vi "Handle Error.vi"(8 "error in (no error)":errorcluster, 11 "UI ActorTop in":refnum<class "CallActorCenter.lvclass">) -> (0 "error out":errorcluster, 2 "stop actor?":bool=TRUE, 3 "UI ActorTop out":refnum<class "CallActorCenter.lvclass">)   [LabVIEW 2021, in "CallActorCenter.lvclass"]
doc: "(<B>Filename</B>: Actor Framework.lvlib:Actor.lvclass:Handle Error.vi)\n\nDefines how the actor handles an error that occurred while processing a message. By default, this method does nothing except stop the actor."
uses:
  CallActorCenter.lvclass
  C:/Program Files (x86)/National Instruments/LabVIEW 2021/user.lib/John_Lib/AbstractActorTemplate/AbstractActorTemplate/UIActorTop.lvclass
  <vilib>/ActorFramework/Stop Msg/Stop Msg.lvclass/Stop Msg.ctl
  <vilib>/ActorFramework/Message Enqueuer/Message Enqueuer.lvclass/Message Enqueuer.ctl
  <vilib>/ActorFramework/Message Enqueuer/Enqueue Critical.vi
  <vilib>/ActorFramework/Stop Msg/Stop Msg.lvclass
  C:/Program Files (x86)/National Instruments/LabVIEW 2021/vi.lib/ActorFramework/Message/Message.lvclass
  <vilib>/ActorFramework/Message Priority Queue/Priority Enqueue.vi
  <userlib>/John_Lib/AbstractActorTemplate/AbstractActorTemplate/UIActorTop.lvclass
  <vilib>/ActorFramework/Message Enqueuer/Message Enqueuer.lvclass
  CallActorCenter.lvclass/CallActorCenter.ctl
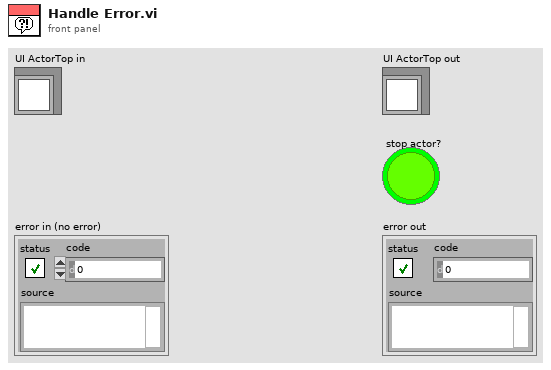
[diagram p1: front panel]
types:
  T1 = map{string, refnum<class "Message Enqueuer.lvclass">}
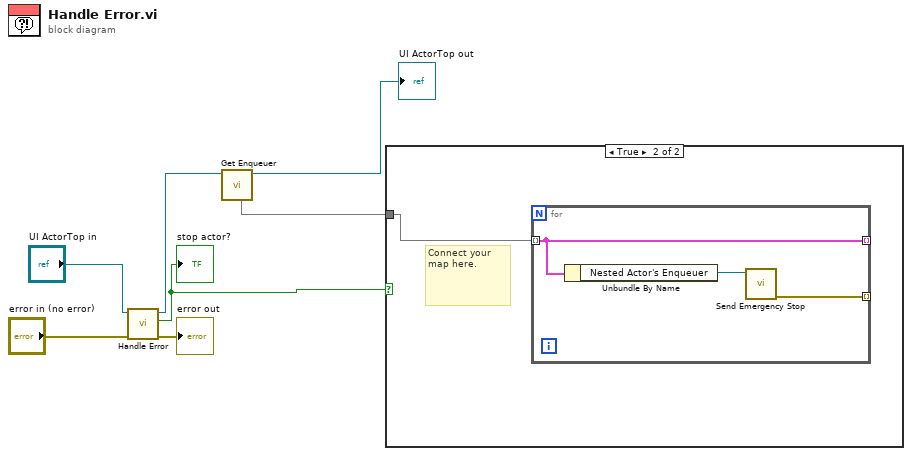
[diagram p0: block diagram]
diagram:
  n1 = call-parent "Handle Error.vi"("error in (no error)"="error in (no error)", "UI ActorTop in"="UI ActorTop in") -> ("error out"=→"error out":errorcluster, "stop actor?"=w4:bool, "UI ActorTop out"=w3:refnum<class "CallActorCenter.lvclass">)  [unwired: 7 in]
  "stop actor?" <- w4
  n2 = call <userlib>:"Get Enqueuer.vi"("UIActorTop in"=w3) -> ("UIActorTop out"=→"UI ActorTop out":refnum<class "CallActorCenter.lvclass">, "Enqueuer"=w2:T1)  [unwired: 6 in, 3 out]
  n3 = case shown="True" w4 {
    tunnel: w2 -> [_ w8]
    frame False {
    }
    frame True {
      # "Connect your map here."
      n4 = for {
        tunnel: [w11] -> _ mode=indexing
        tunnel: w8 -> [w11] mode=indexing
        tunnel: [w9] -> _ mode=indexing
        n5 = Unbundle By Name(w11) -> ("Nested Actor's Enqueuer"=w10:refnum<class "Message Enqueuer.lvclass">)
        n6 = call <vilib>:"Send Emergency Stop.vi"("Message Enqueuer"=w10) -> ("error out"=w9:errorcluster)  [unwired: 10 in]
      }
    }
  }
